vi "nth Derivative of Rational Polynomial (DBL).vi"(9 "order":i32, 10 "Q(x)":dbl[](array[numeric]) min=0.0 max=127.0 format="%#.2g", 11 "P(x)":dbl[](array[numeric]) min=0.0 max=127.0 format="%#.2g") -> (0 "error":i32, 2 "Denominator d[P(x)/Q(x)]/dx":dbl[](array[numeric]) min=0.0 max=127.0 format="%#.2g", 3 "Numerator d[P(x)/Q(x)]/dx":dbl[](array[numeric]) min=0.0 max=127.0 format="%#.2g")   [LabVIEW 2020, in "NI_AALPro.lvlib"]
doc: "Calculates the nth order derivative of a rational polynomial. The data types you wire to the <B>P(x)</B> and <B>Q(x)</B> inputs determine the polymorphic instance to use."
uses:
  NI_AALPro.lvlib
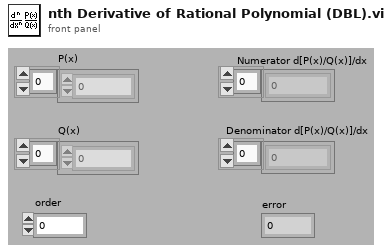
[diagram p1: front panel]
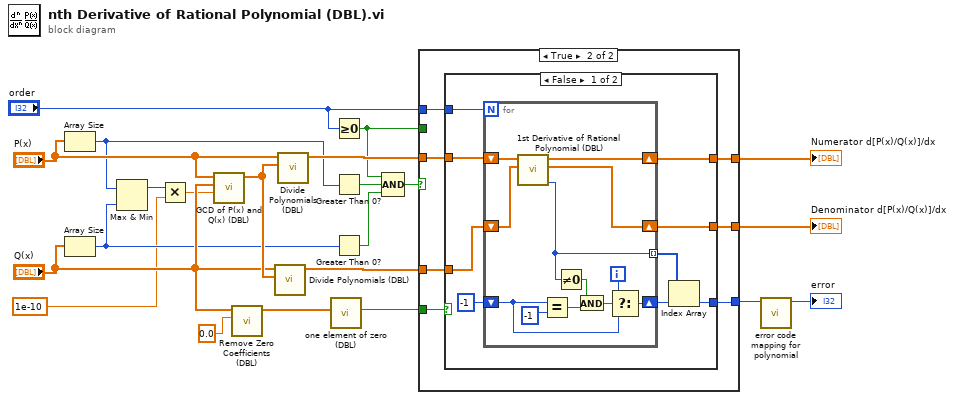
[diagram p0: block diagram]
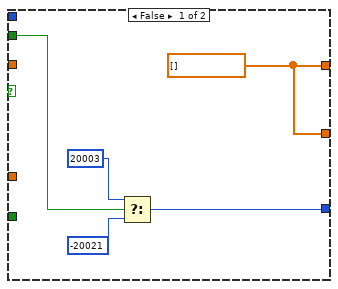
[diagram p2: hidden frame]
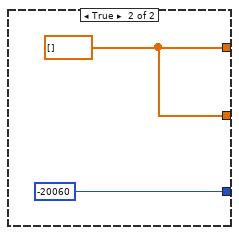
[diagram p3: hidden frame]
diagram:
  n1 = Array Size(array="P(x)") -> (size(s)=w9:i32)
  n2 = Array Size(array="Q(x)") -> (size(s)=w8:i32)
  n3 = Max & Min(x=w9, y=w8) -> (max(x,y)=w10:i32)  [unwired: 1 out]
  n4 = Multiply(x=w10, y=1e-10 ("eps for nth div of p/q")) -> (x*y=w3:dbl)
  n5 = call "GCD of P(x) and Q(x) (DBL).vi"("tolerance"=w3, "Q(x)"="Q(x)", "P(x)"="P(x)") -> ("Greatest Common Divisor"=w14:dbl[])  [unwired: 7 in, 1 out]
  n6 = call "Remove Zero Coefficients (DBL).vi"("threshold"=0.0, "P(x) In"="Q(x)") -> ("P(x) Out"=w6:dbl[])  [unwired: 7 in, 2 out]
  n7 = call "Divide Polynomials (DBL).vi"("Q(x)"=w14, "P(x)"="Q(x)") -> ("P(x)/Q(x)"=w13:dbl[])  [unwired: 7 in, 2 out]
  n8 = call "Divide Polynomials (DBL).vi"("Q(x)"=w14, "P(x)"="P(x)") -> ("P(x)/Q(x)"=w22:dbl[])  [unwired: 7 in, 2 out]
  n9 = call "one element of zero (DBL).vi"("Array in"=w6) -> ("equal [0]?"=w5:bool)  [unwired: 10 in]
  n10 = Greater Or Equal To 0?(x="order") -> (x >= 0?=w4:bool)
  n11 = Greater Than 0?(x=w9) -> (x > 0?=w17:bool)
  n12 = Greater Than 0?(x=w8) -> (x > 0?=w16:bool)
  n13 = Compound Arithmetic op=AND(w4, w17, w16) -> (w15:bool)
  n14 = case shown="True" w15 {
    tunnel: w22 -> [_ w34]
    tunnel: "order" -> [_ w30]
    tunnel: [w27 w33] -> w21
    tunnel: w13 -> [_ w32]
    tunnel: [w27 w31] -> w20
    tunnel: w5 -> [_ w29]
    tunnel: w4 -> [w26 _]
    tunnel: [w23 w28] -> w2
    frame False {
      w27 = dbl[] [] ("Numerator d[p(s)/q(s)]/ds")
      n15 = Select(t=20003 ("empty array"), s=w26, f=-20021 ("minus order")) -> (s? t:f=w23:i32)
    }
    frame True {
      n16 = case shown="False" w29 {
        tunnel: w34 -> [w43 _]
        tunnel: [w42 w57] -> w33
        tunnel: w32 -> [w41 _]
        tunnel: [w40 w57] -> w31
        tunnel: w30 -> [w39 _]
        tunnel: [w35 -20060 ("divide by zero")] -> w28
        frame False {
          n17 = for {
            N: w39 -> [_]
            shift-right: [w53] -> w42
            shift-left: w43 -> [w55]
            shift-right: [w52] -> w40
            shift-left: w41 -> [w54]
            shift-right: [w47] -> w37
            shift-left: -1 -> [w46]
            tunnel: [w44] -> w36 mode=indexing
            i -> [w45]
            n18 = call "1st Derivative of Rational Polynomial (DBL).vi"("Q(x)"=w54, "P(x)"=w55) -> ("error"=w44:i32, "Denominator d[P(x)/Q(x)]/dx"=w52:dbl[], "Numerator d[P(x)/Q(x)]/dx"=w53:dbl[])  [unwired: 7 in]
            n19 = Equal?(x=w46, y=-1) -> (x = y?=w49:bool)
            n20 = Not Equal To 0?(x=w44) -> (x != 0?=w50:bool)
            n21 = And(x=w50, y=w49) -> (x .and. y?=w48:bool)
            n22 = Select(t=w45, s=w48, f=w46) -> (s? t:f=w47:i32)
          }
          n23 = Index Array(array=w36, index=w37) -> (element=w35:i32)
        }
        frame True {
          w57 = dbl[] [] ("Numerator d[p(s)/q(s)]/ds")
        }
      }
    }
  }
  "Denominator d[P(x)/Q(x)]/dx" <- w20
  "Numerator d[P(x)/Q(x)]/dx" <- w21
  n24 = call "error code mapping for polynomial.vi"("error in"=w2) -> ("error out"=→"error":i32)  [unwired: 10 in]
